vi "Write Field.vi"(7 "field name":string, 8 "error in (no error)":errorcluster, 10 "value":variant, 11 "Value in":refnum<class "Value.lvclass">) -> (0 "error out":errorcluster, 2 "value out":variant, 3 "Value out":refnum<class "Value.lvclass">)   [LabVIEW 2020, in "Value.lvlib" / "Value.lvclass"]
uses:
  Value.lvclass
  cceb9e4b-eb75-48e8-aa55-ce9bdc72e988.vi
  a45a0ea4-a1a3-4c44-a2d0-bd9ac2191226.vi
  c2285a35-9ffd-4e7b-9c27-aea24fb1581d.vi
  8f9649cc-7f21-4ef7-860a-133741f03507.vi
  9a7adfbc-dfd7-46c4-b075-4f0440b83174.vi
  f3df2b06-57d5-4a32-8a6e-a93eab4b8334.vi
  1bea9b6c-c326-4b2e-8e3d-45bf733a9c38.vi
  e383973c-90af-4a51-a4c7-5bbe8c763ef6.vi
  d9fbc47b-4e38-408d-93dd-f03e8c927dfc.vi
  f8e0b90b-c4e6-43ce-b49d-bcdb382c13bb.vi
  878da8d4-af84-4ac8-b8bd-4e3d6f536ca0.vi
  1aa6b969-7b68-4eb2-b836-e13a600a071e.vi
  22b99ade-ebf6-47b9-88b0-a2a84584e77c.vi
  0ecc3a10-4d88-4a3f-8e2b-6d81b1eb2788.vi
  7938dc55-06bb-4f46-98b4-31ec94e48f5a.vi
  9cf4c5a1-706a-4248-a3ee-b4c9f4ce04b3.vi
  17bcbbb4-445b-4ae2-9ca0-bb438421ceb4.vi
  ae889fb9-670a-49f8-b5e5-a0c16fe27676.vi
  76e53dd5-f0c3-4a89-968d-82371d9cf6ec.vi
  bc742d90-07da-41a2-bb0a-7e7b2f4baedd.vi
  9c6bba7f-697c-4d5e-a550-b75ffba85a50.vi
  d17b89b1-25de-4b77-9841-199634659aba.vi
  02c85caf-8b62-432b-a175-5fdc5c038fcc.vi
  db2778e5-0a0b-476e-a616-76c34d6078df.vi
  5a5bdb7c-77ef-45fb-97e8-dbe02cadd076.vi
  03112d84-5c9b-4772-aceb-1428f387a576.vi
  b370053f-91cb-4be5-8525-cb241afcd6fe.vi
  21acc165-9bb3-46db-a53e-93d4eb7e31ab.vi
  a549df2c-920d-4323-ba7c-d4da420400e8.vi
  6d74252b-ad3a-45a7-9484-b3c05cdeac0b.vi
  79192ce2-8dd6-4a70-8822-a4eb65a6aaee.vi
  8a659153-4bf4-400b-b716-4e15b1f2a15f.vi
  1431eaa6-23a1-45b9-a4a3-2693041a1402.vi
  8366b1b6-5195-4a32-8846-ef1dc1edc039.vi
  05adf883-15cd-45cb-9d7e-7746134da8fa.vi
  522d9441-c019-479c-9fbf-718d84229053.vi
  2414d7e0-05f5-4190-ab07-d4c7ba67c6a6.vi
  16fc2f7d-2f3d-48d7-828e-6f1655900f08.vi
  efa8a1d7-3bed-4705-901c-3918d28cffa5.vi
  be3d0229-b834-4748-a57b-b2038c1c1ccb.vi
  26f11cd7-ec94-4004-9a33-110acaed2e3e.vi
  270ebb12-d336-49d8-bcbc-e0196ad89af1.vi
  cc62e3b5-8986-4e79-a38c-535dac47f5c9.vi
  6a645410-e7ef-4ed8-b58d-cdb6402696f2.vi
  21c48d27-f92c-4ff3-9f7e-da22303d9520.vi
  71c37fb2-0984-443b-b7b1-928344430237.vi
  0dfc8336-85bc-4349-aa6f-77eea7d3ae68.vi
  d4fece01-f7e1-4bf9-a8a9-9bacda043edb.vi
  <vilib>/Utility/error.llb/Clear Errors.vi
  <vilib>/Utility/Data Type/Get Type Information.vi
  <vilib>/Utility/Data Type/Get Array Information.vi
  <vilib>/Utility/error.llb/Error Cluster From Error Code.vi
  Get Library Path.vi
  <vilib>/ErrorRing/Error Ring.xnode
  Value.lvlib
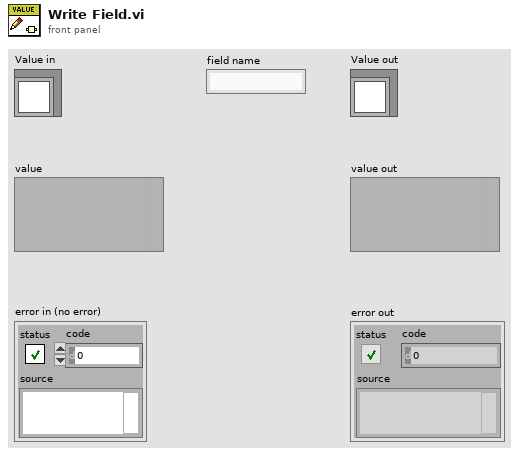
[diagram p1: front panel]
types:
  T1 = typedef "Value.lvlib/Type Code.ctl" = enum8{"Null", "Bool", "BoolA", "Int8", "Int8A", "Int16", "Int16A", "Int32", "Int32A", "Int64", "Int64A", "UInt8", "UInt8A", "UInt16", "UInt16A", "UInt32", "UInt32A", "UInt64", "UInt64A", "Float32", "Float32A", "Float64", "Float64A", "String", "StringA", "Struct", "StructA", "Union", "UnionA", "Any", "AnyA"}
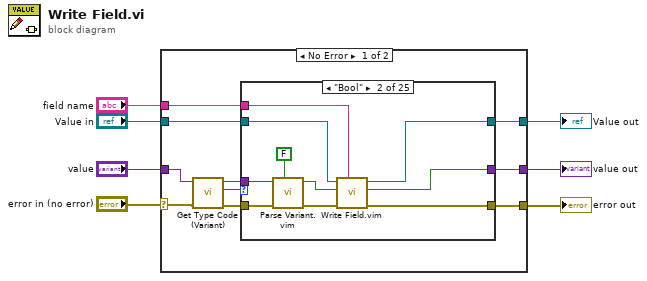
[diagram p0: block diagram]
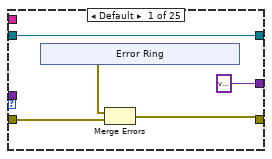
[diagram p2: hidden frame]
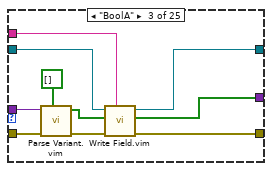
[diagram p3: hidden frame]
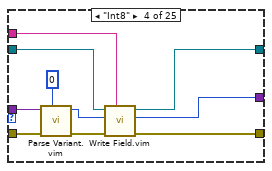
[diagram p4: hidden frame]
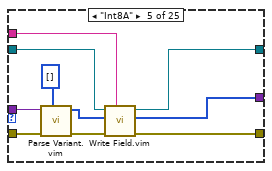
[diagram p5: hidden frame]
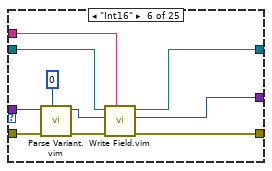
[diagram p6: hidden frame]
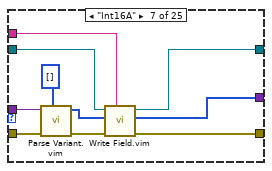
[diagram p7: hidden frame]
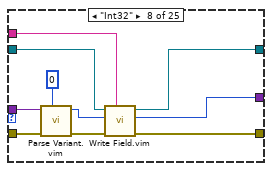
[diagram p8: hidden frame]
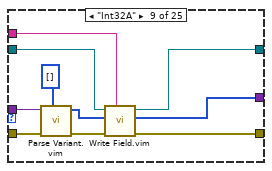
[diagram p9: hidden frame]
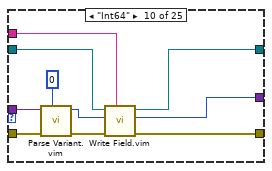
[diagram p10: hidden frame]
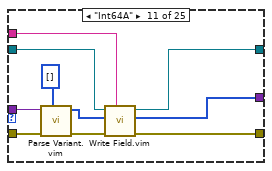
[diagram p11: hidden frame]
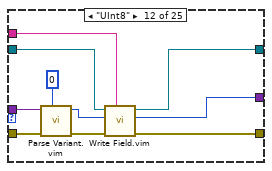
[diagram p12: hidden frame]
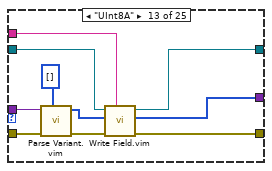
[diagram p13: hidden frame]
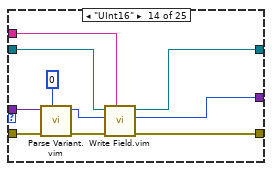
[diagram p14: hidden frame]
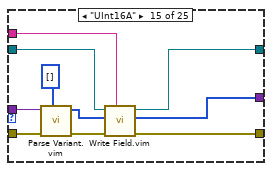
[diagram p15: hidden frame]
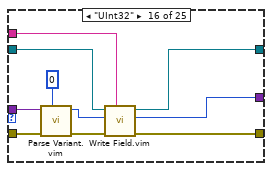
[diagram p16: hidden frame]
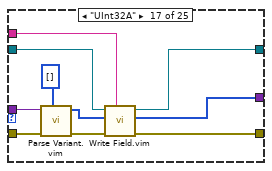
[diagram p17: hidden frame]
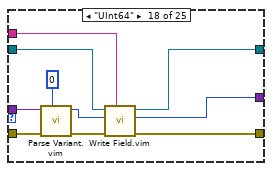
[diagram p18: hidden frame]
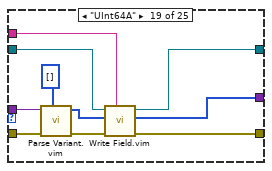
[diagram p19: hidden frame]
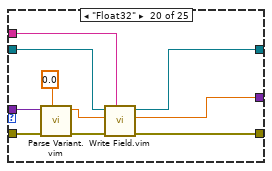
[diagram p20: hidden frame]
diagram:
  n1 = case shown="No Error" "error in (no error)" {
    selector: "error in (no error)" -> [w14 w267]
    tunnel: "value" -> [w13 w268]
    tunnel: [w12 w268] -> w5
    tunnel: [w11 w267] -> w4
    tunnel: "Value in" -> [w10 w269]
    tunnel: [w9 w269] -> w2
    tunnel: "field name" -> [w8 _]
    frame No Error {
      n2 = call "Get Type Code (Variant).vi"("error in (no error)"=w14, "value"=w13) -> ("error out"=w15:errorcluster, "type code"=w17:T1, "value dup"=w16:variant)  [unwired: 5 in]
      n3 = case shown="\"Bool\"" w17 {
        tunnel: [w21 w33 w44 w54 w64 w74 w84 w94 w104 w114 w125 w134 w144 w154 w164 w174 w184 w194 w204 w214 w224 w234 w244 w254 w264] -> w11
        tunnel: w15 -> [w22 w36 w46 w56 w66 w76 w86 w96 w106 w116 w126 w136 w146 w156 w166 w176 w186 w196 w206 w216 w226 w236 w246 w256 w266]
        tunnel: [w18 w31 w42 w53 w62 w72 w82 w92 w102 w112 w123 w132 w142 w153 w162 w172 w183 w192 w202 w212 w222 w232 w242 w252 w262] -> w9
        tunnel: w16 -> [_ w30 w41 w52 w61 w71 w81 w91 w101 w111 w122 w131 w141 w152 w161 w171 w182 w191 w201 w211 w221 w231 w241 w251 w261]
        tunnel: [variant w29 w39 w50 w59 w69 w79 w89 w99 w109 w120 w129 w139 w150 w159 w169 w180 w189 w199 w209 w219 w229 w239 w249 w259] -> w12
        tunnel: w10 -> [w18 w28 w38 w49 w58 w68 w78 w88 w98 w108 w118 w128 w138 w149 w158 w168 w179 w188 w198 w208 w218 w228 w238 w247 w258]
        tunnel: w8 -> [_ w27 w37 w47 w57 w67 w77 w87 w97 w107 w117 w127 w137 w147 w157 w167 w177 w187 w197 w207 w217 w227 w237 w248 w257]
        frame Default {
          n4 = xnode "Error Ring"() -> ("error out"=w20:errorcluster)
          n5 = Merge Errors(w20, w22) -> (w21:errorcluster)
        }
        frame "Bool" {
          n6 = call "Parse Variant.vim"("default"=FALSE, "error in (no error)"=w36, "value"=w30) -> ("error out"=w34:errorcluster, "value out"=w32:bool)  [unwired: 7 in]
          n7 = call "Write Field.vim"("field name"=w27, "error in"=w34, "value"=w32, "Value in"=w28) -> ("error out"=w33:errorcluster, "value out"=w29:bool, "Value out"=w31:refnum<class "Value.lvclass">)  [unwired: 5 in]
        }
        frame "BoolA" {
          n8 = call "Parse Variant.vim"("default"=bool[] [], "error in (no error)"=w46, "value"=w41) -> ("error out"=w45:errorcluster, "value out"=w43:bool[])  [unwired: 7 in]
          n9 = call "Write Field.vim"("field name"=w37, "error in"=w45, "value"=w43, "Value in"=w38) -> ("error out"=w44:errorcluster, "value out"=w39:bool[], "Value out"=w42:refnum<class "Value.lvclass">)  [unwired: 5 in]
        }
        frame "Int8" {
          n10 = call "Parse Variant.vim"("default"=i8 0, "error in (no error)"=w56, "value"=w52) -> ("error out"=w55:errorcluster, "value out"=w48:i8)  [unwired: 7 in]
          n11 = call "Write Field.vim"("field name"=w47, "error in"=w55, "value"=w48, "Value in"=w49) -> ("error out"=w54:errorcluster, "value out"=w50:i8, "Value out"=w53:refnum<class "Value.lvclass">)  [unwired: 5 in]
        }
        frame "Int8A" {
          n12 = call "Parse Variant.vim"("default"=i8[] [], "error in (no error)"=w66, "value"=w61) -> ("error out"=w65:errorcluster, "value out"=w63:i8[])  [unwired: 7 in]
          n13 = call "Write Field.vim"("field name"=w57, "error in"=w65, "value"=w63, "Value in"=w58) -> ("error out"=w64:errorcluster, "value out"=w59:i8[], "Value out"=w62:refnum<class "Value.lvclass">)  [unwired: 5 in]
        }
        frame "Int16" {
          n14 = call "Parse Variant.vim"("default"=i16 0, "error in (no error)"=w76, "value"=w71) -> ("error out"=w75:errorcluster, "value out"=w73:i16)  [unwired: 7 in]
          n15 = call "Write Field.vim"("field name"=w67, "error in"=w75, "value"=w73, "Value in"=w68) -> ("error out"=w74:errorcluster, "value out"=w69:i16, "Value out"=w72:refnum<class "Value.lvclass">)  [unwired: 5 in]
        }
        frame "Int16A" {
          n16 = call "Parse Variant.vim"("default"=i16[] [], "error in (no error)"=w86, "value"=w81) -> ("error out"=w85:errorcluster, "value out"=w83:i16[])  [unwired: 7 in]
          n17 = call "Write Field.vim"("field name"=w77, "error in"=w85, "value"=w83, "Value in"=w78) -> ("error out"=w84:errorcluster, "value out"=w79:i16[], "Value out"=w82:refnum<class "Value.lvclass">)  [unwired: 5 in]
        }
        frame "Int32" {
          n18 = call "Parse Variant.vim"("default"=0, "error in (no error)"=w96, "value"=w91) -> ("error out"=w95:errorcluster, "value out"=w93:i32)  [unwired: 7 in]
          n19 = call "Write Field.vim"("field name"=w87, "error in"=w95, "value"=w93, "Value in"=w88) -> ("error out"=w94:errorcluster, "value out"=w89:i32, "Value out"=w92:refnum<class "Value.lvclass">)  [unwired: 5 in]
        }
        frame "Int32A" {
          n20 = call "Parse Variant.vim"("default"=i32[] [], "error in (no error)"=w106, "value"=w101) -> ("error out"=w105:errorcluster, "value out"=w103:i32[])  [unwired: 7 in]
          n21 = call "Write Field.vim"("field name"=w97, "error in"=w105, "value"=w103, "Value in"=w98) -> ("error out"=w104:errorcluster, "value out"=w99:i32[], "Value out"=w102:refnum<class "Value.lvclass">)  [unwired: 5 in]
        }
        frame "Int64" {
          n22 = call "Parse Variant.vim"("default"=i64 0, "error in (no error)"=w116, "value"=w111) -> ("error out"=w115:errorcluster, "value out"=w113:i64)  [unwired: 7 in]
          n23 = call "Write Field.vim"("field name"=w107, "error in"=w115, "value"=w113, "Value in"=w108) -> ("error out"=w114:errorcluster, "value out"=w109:i64, "Value out"=w112:refnum<class "Value.lvclass">)  [unwired: 5 in]
        }
        frame "Int64A" {
          n24 = call "Parse Variant.vim"("default"=i64[] [], "error in (no error)"=w126, "value"=w122) -> ("error out"=w119:errorcluster, "value out"=w124:i64[])  [unwired: 7 in]
          n25 = call "Write Field.vim"("field name"=w117, "error in"=w119, "value"=w124, "Value in"=w118) -> ("error out"=w125:errorcluster, "value out"=w120:i64[], "Value out"=w123:refnum<class "Value.lvclass">)  [unwired: 5 in]
        }
        frame "UInt8" {
          n26 = call "Parse Variant.vim"("default"=u8 0, "error in (no error)"=w136, "value"=w131) -> ("error out"=w135:errorcluster, "value out"=w133:u8)  [unwired: 7 in]
          n27 = call "Write Field.vim"("field name"=w127, "error in"=w135, "value"=w133, "Value in"=w128) -> ("error out"=w134:errorcluster, "value out"=w129:u8, "Value out"=w132:refnum<class "Value.lvclass">)  [unwired: 5 in]
        }
        frame "UInt8A" {
          n28 = call "Parse Variant.vim"("default"=u8[] [], "error in (no error)"=w146, "value"=w141) -> ("error out"=w145:errorcluster, "value out"=w143:u8[])  [unwired: 7 in]
          n29 = call "Write Field.vim"("field name"=w137, "error in"=w145, "value"=w143, "Value in"=w138) -> ("error out"=w144:errorcluster, "value out"=w139:u8[], "Value out"=w142:refnum<class "Value.lvclass">)  [unwired: 5 in]
        }
        frame "UInt16" {
          n30 = call "Parse Variant.vim"("default"=u16 0, "error in (no error)"=w156, "value"=w152) -> ("error out"=w155:errorcluster, "value out"=w148:u16)  [unwired: 7 in]
          n31 = call "Write Field.vim"("field name"=w147, "error in"=w155, "value"=w148, "Value in"=w149) -> ("error out"=w154:errorcluster, "value out"=w150:u16, "Value out"=w153:refnum<class "Value.lvclass">)  [unwired: 5 in]
        }
        frame "UInt16A" {
          n32 = call "Parse Variant.vim"("default"=u16[] [], "error in (no error)"=w166, "value"=w161) -> ("error out"=w165:errorcluster, "value out"=w163:u16[])  [unwired: 7 in]
          n33 = call "Write Field.vim"("field name"=w157, "error in"=w165, "value"=w163, "Value in"=w158) -> ("error out"=w164:errorcluster, "value out"=w159:u16[], "Value out"=w162:refnum<class "Value.lvclass">)  [unwired: 5 in]
        }
        frame "UInt32" {
          n34 = call "Parse Variant.vim"("default"=u32 0, "error in (no error)"=w176, "value"=w171) -> ("error out"=w175:errorcluster, "value out"=w173:u32)  [unwired: 7 in]
          n35 = call "Write Field.vim"("field name"=w167, "error in"=w175, "value"=w173, "Value in"=w168) -> ("error out"=w174:errorcluster, "value out"=w169:u32, "Value out"=w172:refnum<class "Value.lvclass">)  [unwired: 5 in]
        }
        frame "UInt32A" {
          n36 = call "Parse Variant.vim"("default"=u32[] [], "error in (no error)"=w186, "value"=w182) -> ("error out"=w185:errorcluster, "value out"=w178:u32[])  [unwired: 7 in]
          n37 = call "Write Field.vim"("field name"=w177, "error in"=w185, "value"=w178, "Value in"=w179) -> ("error out"=w184:errorcluster, "value out"=w180:u32[], "Value out"=w183:refnum<class "Value.lvclass">)  [unwired: 5 in]
        }
        frame "UInt64" {
          n38 = call "Parse Variant.vim"("default"=u64 0, "error in (no error)"=w196, "value"=w191) -> ("error out"=w195:errorcluster, "value out"=w193:u64)  [unwired: 7 in]
          n39 = call "Write Field.vim"("field name"=w187, "error in"=w195, "value"=w193, "Value in"=w188) -> ("error out"=w194:errorcluster, "value out"=w189:u64, "Value out"=w192:refnum<class "Value.lvclass">)  [unwired: 5 in]
        }
        frame "UInt64A" {
          n40 = call "Parse Variant.vim"("default"=u64[] [], "error in (no error)"=w206, "value"=w201) -> ("error out"=w205:errorcluster, "value out"=w203:u64[])  [unwired: 7 in]
          n41 = call "Write Field.vim"("field name"=w197, "error in"=w205, "value"=w203, "Value in"=w198) -> ("error out"=w204:errorcluster, "value out"=w199:u64[], "Value out"=w202:refnum<class "Value.lvclass">)  [unwired: 5 in]
        }
        frame "Float32" {
          n42 = call "Parse Variant.vim"("default"=sgl 0.0, "error in (no error)"=w216, "value"=w211) -> ("error out"=w215:errorcluster, "value out"=w213:sgl)  [unwired: 7 in]
          n43 = call "Write Field.vim"("field name"=w207, "error in"=w215, "value"=w213, "Value in"=w208) -> ("error out"=w214:errorcluster, "value out"=w209:sgl, "Value out"=w212:refnum<class "Value.lvclass">)  [unwired: 5 in]
        }
        frame "Float64" {
          n44 = call "Parse Variant.vim"("default"=0.0, "error in (no error)"=w226, "value"=w221) -> ("error out"=w225:errorcluster, "value out"=w223:dbl)  [unwired: 7 in]
          n45 = call "Write Field.vim"("field name"=w217, "error in"=w225, "value"=w223, "Value in"=w218) -> ("error out"=w224:errorcluster, "value out"=w219:dbl, "Value out"=w222:refnum<class "Value.lvclass">)  [unwired: 5 in]
        }
        frame "Float32A" {
          n46 = call "Parse Variant.vim"("default"=sgl[] [], "error in (no error)"=w236, "value"=w231) -> ("error out"=w235:errorcluster, "value out"=w233:sgl[])  [unwired: 7 in]
          n47 = call "Write Field.vim"("field name"=w227, "error in"=w235, "value"=w233, "Value in"=w228) -> ("error out"=w234:errorcluster, "value out"=w229:sgl[], "Value out"=w232:refnum<class "Value.lvclass">)  [unwired: 5 in]
        }
        frame "Float64A" {
          n48 = call "Parse Variant.vim"("default"=dbl[] [], "error in (no error)"=w246, "value"=w241) -> ("error out"=w245:errorcluster, "value out"=w243:dbl[])  [unwired: 7 in]
          n49 = call "Write Field.vim"("field name"=w237, "error in"=w245, "value"=w243, "Value in"=w238) -> ("error out"=w244:errorcluster, "value out"=w239:dbl[], "Value out"=w242:refnum<class "Value.lvclass">)  [unwired: 5 in]
        }
        frame "String" {
          n50 = call "Parse Variant.vim"("default"="", "error in (no error)"=w256, "value"=w251) -> ("error out"=w255:errorcluster, "value out"=w253:string)  [unwired: 7 in]
          n51 = call "Write Field.vim"("field name"=w248, "error in"=w255, "value"=w253, "Value in"=w247) -> ("error out"=w254:errorcluster, "value out"=w249:string, "Value out"=w252:refnum<class "Value.lvclass">)  [unwired: 5 in]
        }
        frame "StringA" {
          n52 = call "Parse Variant.vim"("default"=string[] [], "error in (no error)"=w266, "value"=w261) -> ("error out"=w265:errorcluster, "value out"=w263:string[])  [unwired: 7 in]
          n53 = call "Write Field.vim"("field name"=w257, "error in"=w265, "value"=w263, "Value in"=w258) -> ("error out"=w264:errorcluster, "value out"=w259:string[], "Value out"=w262:refnum<class "Value.lvclass">)  [unwired: 5 in]
        }
      }
    }
    frame Error {
    }
  }
  "value out" <- w5
  "error out" <- w4
  "Value out" <- w2
